vi "Action 1.vi"(8 "error in (no error)":errorcluster, 11 "Interface 3 in":refnum<class "IconEditor.lvclass">) -> (0 "error out":errorcluster, 3 "Interface 3 out":refnum<class "IconEditor.lvclass">)   [LabVIEW 2021, in "lv_icon.lvlib" / "IconEditor.lvclass"]
uses:
  <vilib>/LabVIEW Icon API/lv_icon/Interface 3/IconEditor.lvclass
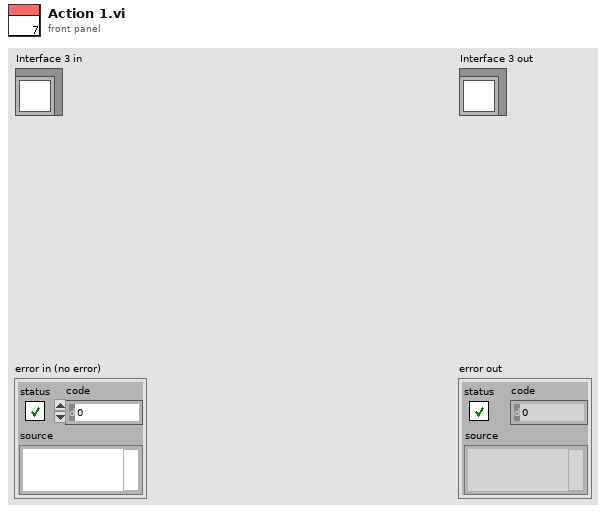
[diagram p1: front panel]
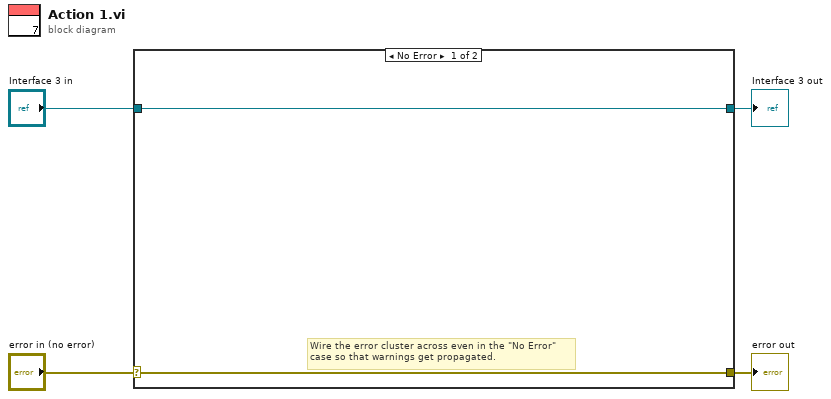
[diagram p0: block diagram]
diagram:
  n1 = case shown="No Error" "error in (no error)" {
    selector: "error in (no error)" -> [w5 w8]
    tunnel: [w5 w8] -> w3
    tunnel: [w6 w7] -> w1
    tunnel: "Interface 3 in" -> [w6 w7]
    frame No Error {
      # "Wire the error cluster across even in the \"No Error\"\ncase so that warnings get propagated."
    }
    frame Error {
    }
  }
  "error out" <- w3
  "Interface 3 out" <- w1
